vi "GOOP_TimeDebug.vi"(10 "Flag":string) -> ()   [LabVIEW 2016]
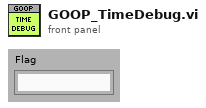
[diagram p1: front panel]
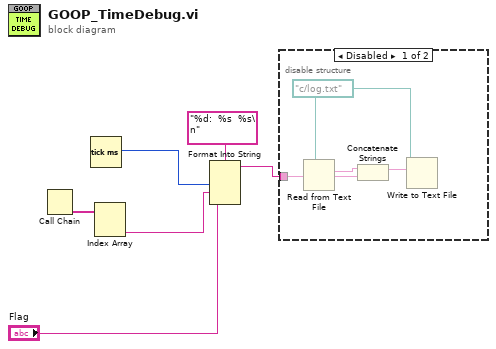
[diagram p0: block diagram]
diagram:
  n1 = Call Chain() -> (call chain=w6:string[])
  n2 = Tick Count (ms)() -> (millisecond timer value=w5:u32)
  n3 = Index Array(array=w6) -> (element #2=w3:string)  [unwired: 2 in, 1 out]
  n4 = Format Into String(format string="%d:  %s  %s\n", w5, w3, "Flag") -> (resulting string=w2:string)  [unwired: 2 in, 1 out]
  n5 = disable-structure shown="Disabled" {
    disable-tunnel: w2 -> [w9 _]
    frame Disabled {
      w7 = path "c:/log.txt" ("file (use dialog)")
      n6 = Read from Text File(file (use dialog)=w7) -> (text=w10:string)  [unwired: 3 in, 3 out]
      n7 = Concatenate Strings(w10, w9) -> (w8:string)
      n8 = Write to Text File(file (use dialog)=w7, text=w8) -> ()  [unwired: 2 in, 3 out]
    }
    frame Enabled {
    }
  }
